vi "Thread@Thread Stop__Parameter.vi"(1 "ParamterIn":string) -> (0 "ParamterOut":string)   [LabVIEW 2020]
panel:
  in  "ErrorMessage":string(combo)
  in  "Logic":string(combo)
  in  "Confirm":bool
  # "Thread@Thread Stop ($Logic,$ErrorMessage)"
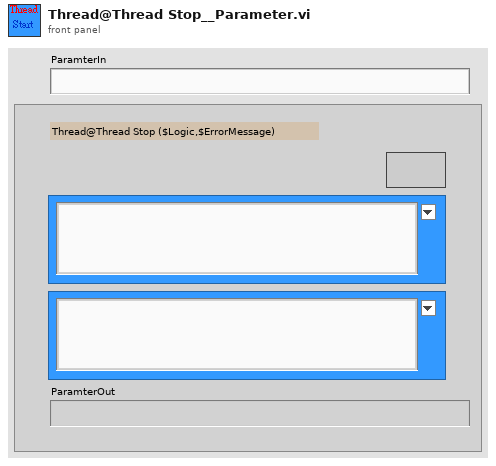
[diagram p1: front panel]
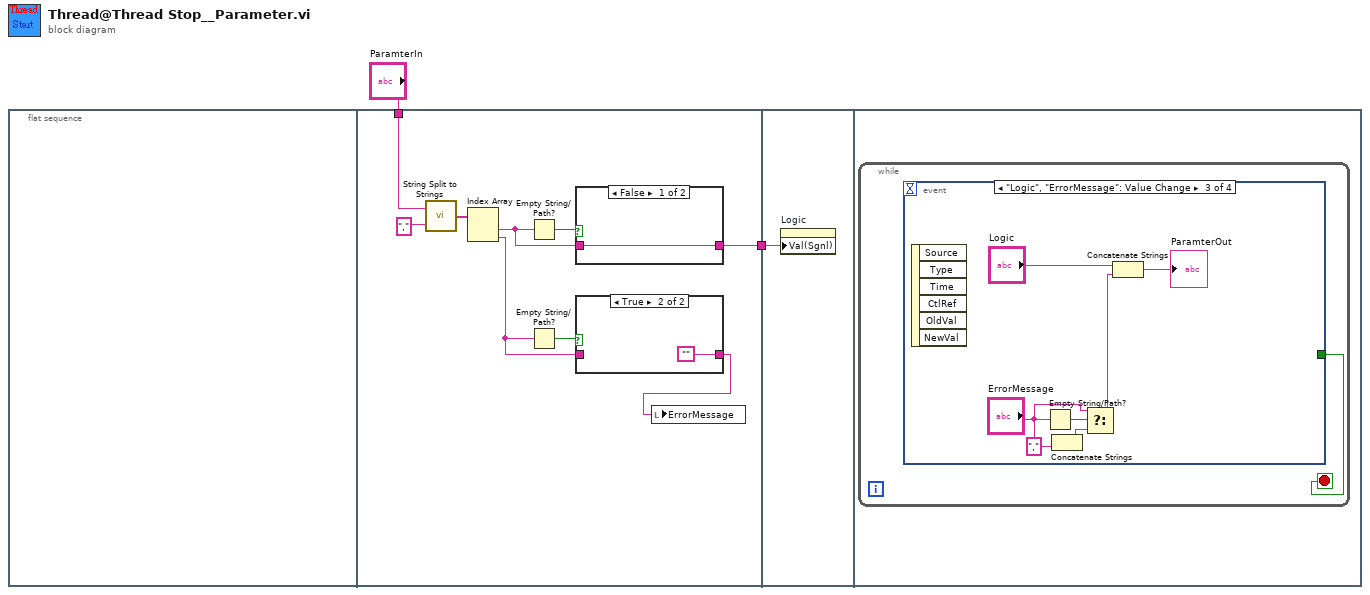
[diagram p0: block diagram]
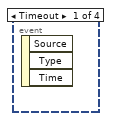
[diagram p4: hidden frame]
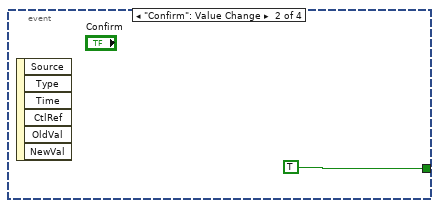
[diagram p5: hidden frame]
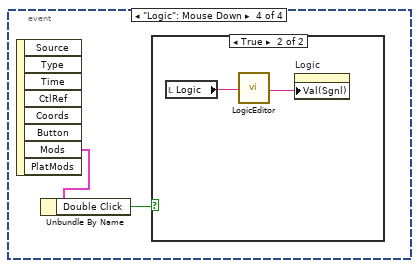
[diagram p6: hidden frame]
diagram:
  n1 = flat-sequence {
    tunnel: "ParamterIn" -> [w9]
    tunnel: [w6] -> w1
    tunnel: w1 -> [w15]
    frame #0 {
    }
    frame #1 {
      n2 = call "String Split to Strings.vi"("search string/char (-)"=",", "String"=w9) -> ("Array"=w11:string[])
      n3 = Index Array(array=w11) -> (element #1=w7:string, element #2=w4:string)  [unwired: 2 in]
      n4 = Empty String/Path?(string/path=w7) -> (empty?=w8:bool)
      n5 = Empty String/Path?(string/path=w4) -> (empty?=w5:bool)
      n6 = case shown="False" w8 {
        tunnel: w7 -> [w14 _]
        tunnel: [w14 _] -> w6
        frame False {
        }
        frame True {
        }
      }
      n7 = case shown="True" w5 {
        tunnel: w4 -> [w12 _]
        tunnel: [w12 ""] -> w3
        frame False {
        }
        frame True {
        }
      }
      n8 = local write "ErrorMessage"(w3) -> ()
    }
    frame #2 {
      n9 = property on="Logic" class="CmbBox"("Val(Sgnl)"=w15) -> ()  [unwired: 2 in, 2 out]
    }
    frame #3 {
      n10 = while {
        stop <- w16 stop-if-true
        n11 = event shown="[2] \"Logic\", \"ErrorMessage\": Value Change" {
          selector: _ -> [_ _ _ _]
          dyn-events: _ -> [_ _ _ _]
          timeout: _ -> [_ _ _ _]
          tunnel: [_ TRUE _ _] -> w16
          event Timeout {
            n12 = event-data() -> ()  [unwired: 1 in, 3 out]
          }
          event "Confirm": Value Change {
            n13 = event-data() -> ()  [unwired: 1 in, 6 out]
          }
          event "Logic", "ErrorMessage": Value Change {
            n14 = event-data() -> ()  [unwired: 1 in, 6 out]
            n15 = Empty String/Path?(string/path="ErrorMessage") -> (empty?=w22:bool)
            n16 = Concatenate Strings("," ("string"), "ErrorMessage") -> (w19:string)
            n17 = Select(t="ErrorMessage", s=w22, f=w19) -> (s? t:f=w18:string)
            n18 = Concatenate Strings("Logic", w18) -> (→"ParamterOut":string)
          }
          event "Logic": Mouse Down {
            n19 = event-data() -> ("Mods"=w26:cluster{"Double Click":bool, "Menu Key":bool})  [unwired: 1 in, 7 out]
            n20 = Unbundle By Name(w26) -> ("Double Click"=w25:bool)
            n21 = case shown="True" w25 {
              frame False {
              }
              frame True {
                n22 = local read "Logic"() -> (w28:string)
                n23 = call "LogicEditor.vi"("Logic Express"=w28) -> ("LogicExpressOut"=w27:string)
                n24 = property on="Logic" class="CmbBox"("Val(Sgnl)"=w27) -> ()  [unwired: 2 in, 2 out]
              }
            }
          }
        }
      }
    }
  }
